vi "Process Single Cell in Map.vi"(9 "Step":i32, 10 "Cell":T1, 11 "Map in":map{T1, T2}(c390)) -> (2 "Check Surroundings?":bool, 3 "Map out":map{T1, T2}(c390))   [LabVIEW 2019, in "Grassfire Algorithm.lvclass"]
uses:
  Grassfire Algorithm.lvclass
  Index Column Row--cluster.ctl
  Solution Grid Cell Private--cluster.ctl
  Solution--picture ring.ctl
  Selection--enum.ctl
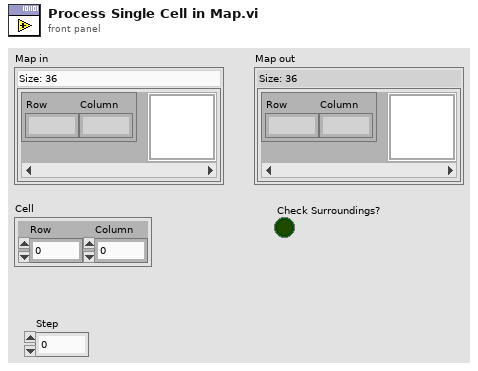
[diagram p1: front panel]
types:
  T1 = typedef "Grassfire Algorithm.lvclass/Index Column Row--cluster.ctl" = cluster{"Row":i32, "Column":i32}
  T2 = typedef "Grassfire Algorithm.lvclass/Solution Grid Cell Private--cluster.ctl" = cluster{"Picture":T3, "Value":dbl}
  T3 = typedef "Grassfire Algorithm.lvclass/Solution--picture ring.ctl" = i64
  T4 = typedef "Grassfire Algorithm.lvclass/Selection--enum.ctl" = enum16{"Empty", "Blocked", "Start", "End", "Path"}
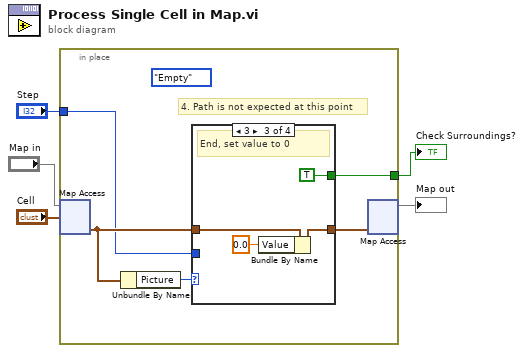
[diagram p0: block diagram]
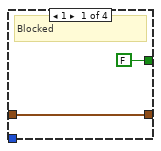
[diagram p2: hidden frame]
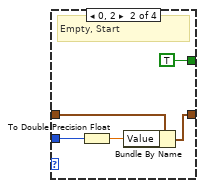
[diagram p3: hidden frame]
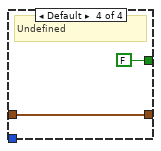
[diagram p4: hidden frame]
diagram:
  n1 = in-place {
    in-place-border: [w7] -> w3
    in-place-border: "Step" -> [w6]
    (unwired) Selection--enum."Empty" ("Selection")
    # "4. Path is not expected at this point"
    n2 = in-place-map #1("Map in", "Cell") -> (w9:T2)  [unwired: 1 in, 1 out]
    n3 = Unbundle By Name(w9) -> ("Picture"=w8:T3)
    n4 = case shown="3" w8 {
      tunnel: [w12 w15 w19 w23] -> w10
      tunnel: w9 -> [w12 w16 w20 w23]
      tunnel: [FALSE TRUE TRUE FALSE] -> w7
      tunnel: w6 -> [_ w14 _ _]
      frame 1 {
        # "Blocked"
      }
      frame 0, 2 {
        # "Empty, Start"
        n5 = To Double Precision Float(number=w14) -> (double precision float=w13:dbl)
        n6 = Bundle By Name(cluster=w16, "Value"=w13) -> (w15:T2)
      }
      frame 3 {
        # "End, set value to 0"
        n7 = Bundle By Name(cluster=w20, "Value"=0.0) -> (w19:T2)
      }
      frame Default {
        # "Undefined"
      }
    }
    n8 = in-place-map #1(w10) -> (→"Map out":map{T1, T2})  [unwired: 1 in, 2 out]
  }
  "Check Surroundings?" <- w3
